vi "Set.vi"(10 "Value":i64, 11 "Integer in":refnum<class "Integer.lvclass">) -> (3 "Integer out":refnum<class "Integer.lvclass">)   [LabVIEW 2022 SP3, in "Conditum.lvlib" / "Columns.lvlib" / "Integer.lvclass"]
uses:
  Integer.lvclass
  C:/dev/lv/illuminated-g/lv-conditum/Conditum/Columns/Type/Type.lvclass
  Type/Type.lvclass/Type.ctl
  Integer.lvclass/Integer.ctl
  Type/Type.lvclass
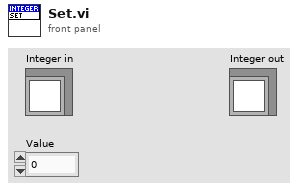
[diagram p1: front panel]
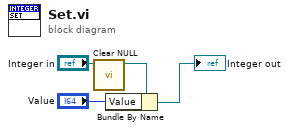
[diagram p0: block diagram]
diagram:
  n1 = call "Clear NULL.vi"("Type in"="Integer in") -> ("Type out"=w1:refnum<class "Integer.lvclass">)  [unwired: 10 in]
  n2 = Bundle By Name(cluster=w1, "Value"="Value") -> (→"Integer out":refnum<class "Integer.lvclass">)
